vi "S4GUI_002.vi"(7 "Tab ObsEng":enum32{"Obs", "CCD modes", "Eng"}(tab)) -> ()   [LabVIEW 2018] (continued)
        n3103 = call-dynamic "Write Suffix.vi"("error in (no error)"=w6685, "Suffix"=w6751, "Interface in"=w6684) -> ("error out"=w6676:errorcluster, "Interface out"=w6679:refnum<class "Interface.lvclass">)  [unwired: 7 in]
        n3104 = call-dynamic "Write Suffix.vi"("error in (no error)"=w6649, "Suffix"=w6751, "Interface in"=w6650) -> ("error out"=w6658:errorcluster, "Interface out"=w6655:refnum<class "Interface.lvclass">)  [unwired: 7 in]
        n3105 = call-dynamic "Write ObsType.vi"("error in (no error)"=w6700, "ObsType"=w6729, "Interface in"=w6704) -> ("error out"=w6701:errorcluster, "Interface out"=w6705:refnum<class "Interface.lvclass">)  [unwired: 7 in]
        n3106 = call-dynamic "Write ObsType.vi"("error in (no error)"=w6624, "ObsType"=w6729, "Interface in"=w6627) -> ("error out"=w6625:errorcluster, "Interface out"=w6628:refnum<class "Interface.lvclass">)  [unwired: 7 in]
        n3107 = call-dynamic "Write ObsType.vi"("error in (no error)"=w6676, "ObsType"=w6729, "Interface in"=w6679) -> ("error out"=w6677:errorcluster, "Interface out"=w6680:refnum<class "Interface.lvclass">)  [unwired: 7 in]
        n3108 = call-dynamic "Write ObsType.vi"("error in (no error)"=w6658, "ObsType"=w6729, "Interface in"=w6655) -> ("error out"=w6657:errorcluster, "Interface out"=w6654:refnum<class "Interface.lvclass">)  [unwired: 7 in]
        n3109 = call-dynamic "Write Object.vi"("error in (no error)"=w6701, "Object"=w6730, "Interface in"=w6705) -> ("error out"=w6702:errorcluster, "Interface out"=w6706:refnum<class "Interface.lvclass">)  [unwired: 7 in]
        n3110 = call-dynamic "Write Object.vi"("error in (no error)"=w6677, "Object"=w6730, "Interface in"=w6680) -> ("error out"=w6678:errorcluster, "Interface out"=w6681:refnum<class "Interface.lvclass">)  [unwired: 7 in]
        n3111 = call-dynamic "Write Object.vi"("error in (no error)"=w6625, "Object"=w6730, "Interface in"=w6628) -> ("error out"=w6626:errorcluster, "Interface out"=w6629:refnum<class "Interface.lvclass">)  [unwired: 7 in]
        n3112 = call-dynamic "Write Object.vi"("error in (no error)"=w6657, "Object"=w6730, "Interface in"=w6654) -> ("error out"=w6656:errorcluster, "Interface out"=w6653:refnum<class "Interface.lvclass">)  [unwired: 7 in]
        n3113 = call-dynamic "Write Comments.vi"("error in (no error)"=w6626, "Comments"=w6723, "Interface in"=w6629) -> ("error out"=w6630:errorcluster, "Interface out"=w6631:refnum<class "Interface.lvclass">)  [unwired: 7 in]
        n3114 = call-dynamic "Write Comments.vi"("error in (no error)"=w6678, "Comments"=w6723, "Interface in"=w6681) -> ("error out"=w6682:errorcluster, "Interface out"=w6683:refnum<class "Interface.lvclass">)  [unwired: 7 in]
        n3115 = call-dynamic "Write Comments.vi"("error in (no error)"=w6656, "Comments"=w6723, "Interface in"=w6653) -> ("error out"=w6652:errorcluster, "Interface out"=w6651:refnum<class "Interface.lvclass">)  [unwired: 7 in]
        n3116 = call-dynamic "Write Comments.vi"("error in (no error)"=w6702, "Comments"=w6723, "Interface in"=w6706) -> ("error out"=w6707:errorcluster, "Interface out"=w6708:refnum<class "Interface.lvclass">)  [unwired: 7 in]
        n3117 = call-dynamic "Write Observer.vi"("error in (no error)"=w6630, "Observer"=w6728, "Interface in"=w6631) -> ("error out"=w6616:errorcluster, "Interface out"=w6615:refnum<class "Interface.lvclass">)  [unwired: 7 in]
        n3118 = call-dynamic "Write Observer.vi"("error in (no error)"=w6707, "Observer"=w6728, "Interface in"=w6708) -> ("error out"=w6693:errorcluster, "Interface out"=w6694:refnum<class "Interface.lvclass">)  [unwired: 7 in]
        n3119 = call-dynamic "Write Observer.vi"("error in (no error)"=w6682, "Observer"=w6728, "Interface in"=w6683) -> ("error out"=w6668:errorcluster, "Interface out"=w6667:refnum<class "Interface.lvclass">)  [unwired: 7 in]
        n3120 = call-dynamic "Write Observer.vi"("error in (no error)"=w6652, "Observer"=w6728, "Interface in"=w6651) -> ("error out"=w6642:errorcluster, "Interface out"=w6641:refnum<class "Interface.lvclass">)  [unwired: 7 in]
        n3121 = call-dynamic "Write Project ID.vi"("error in (no error)"=w6642, "Project ID"=w6727, "Interface in"=w6641) -> ("error out"=w6639:errorcluster, "Interface out"=w6640:refnum<class "Interface.lvclass">)  [unwired: 7 in]
        n3122 = call-dynamic "Write Project ID.vi"("error in (no error)"=w6668, "Project ID"=w6727, "Interface in"=w6667) -> ("error out"=w6665:errorcluster, "Interface out"=w6666:refnum<class "Interface.lvclass">)  [unwired: 7 in]
        n3123 = call-dynamic "Write Project ID.vi"("error in (no error)"=w6616, "Project ID"=w6727, "Interface in"=w6615) -> ("error out"=w6613:errorcluster, "Interface out"=w6614:refnum<class "Interface.lvclass">)  [unwired: 7 in]
        n3124 = call-dynamic "Write Project ID.vi"("error in (no error)"=w6693, "Project ID"=w6727, "Interface in"=w6694) -> ("error out"=w6691:errorcluster, "Interface out"=w6692:refnum<class "Interface.lvclass">)  [unwired: 7 in]
        n3125 = call-dynamic "Write Interface.vi"("error in (no error)"=w6665, "Interface.lvclass"=w6666, "Channel in"=w6674) -> ("error out"=w6672:errorcluster, "Channel out"=w6673:refnum<class "Channel.lvclass">)  [unwired: 7 in]
        n3126 = call-dynamic "Write Interface.vi"("error in (no error)"=w6691, "Interface.lvclass"=w6692, "Channel in"=w6703) -> ("error out"=w6697:errorcluster, "Channel out"=w6698:refnum<class "Channel.lvclass">)  [unwired: 7 in]
        n3127 = call-dynamic "Write Interface.vi"("error in (no error)"=w6639, "Interface.lvclass"=w6640, "Channel in"=w6660) -> ("error out"=w6646:errorcluster, "Channel out"=w6647:refnum<class "Channel.lvclass">)  [unwired: 7 in]
        n3128 = call-dynamic "Write Interface.vi"("error in (no error)"=w6613, "Interface.lvclass"=w6614, "Channel in"=w6622) -> ("error out"=w6620:errorcluster, "Channel out"=w6621:refnum<class "Channel.lvclass">)  [unwired: 7 in]
        n3129 = case shown="True" w6664 {
          tunnel: [w6805 w6816] -> w6689
          tunnel: [w6806 w6815] -> w6688
          tunnel: w6673 -> [w6806 w6808]
          tunnel: w6672 -> [w6805 w6807]
          frame False {
          }
          frame True {
            # "command SET SUFFIX"
            n3130 = call-dynamic "Read State Machine.vi"("error in (no error)"=w6807, "Device in"=w6808) -> ("error out"=w6809:errorcluster, "State Machine.lvclass"=w6813:refnum<class "State Machine.lvclass">, "Device out"=w6812:refnum<class "Channel.lvclass">)  [unwired: 7 in]
            n3131 = call-dynamic "Write State.vi"("error in (no error)"=w6809, "State"=300, "State Machine in"=w6813) -> ("error out"=w6810:errorcluster, "State Machine out"=w6814:refnum<class "State Machine.lvclass">)  [unwired: 7 in]
            n3132 = call-dynamic "Write State Machine.vi"("error in (no error)"=w6810, "State Machine.lvclass"=w6814, "Device in"=w6812) -> ("error out"=w6816:errorcluster, "Device out"=w6815:refnum<class "Channel.lvclass">)  [unwired: 7 in]
          }
        }
        n3133 = case shown="True" w6690 {
          tunnel: [w6818 w6822] -> w6714
          tunnel: [w6817 w6821] -> w6713
          tunnel: w6698 -> [w6818 w6820]
          tunnel: w6697 -> [w6817 w6819]
          frame False {
          }
          frame True {
            # "command SET SUFFIX"
            n3134 = call-dynamic "Read State Machine.vi"("error in (no error)"=w6819, "Device in"=w6820) -> ("error out"=w6828:errorcluster, "State Machine.lvclass"=w6824:refnum<class "State Machine.lvclass">, "Device out"=w6825:refnum<class "Channel.lvclass">)  [unwired: 7 in]
            n3135 = call-dynamic "Write State.vi"("error in (no error)"=w6828, "State"=300, "State Machine in"=w6824) -> ("error out"=w6827:errorcluster, "State Machine out"=w6823:refnum<class "State Machine.lvclass">)  [unwired: 7 in]
            n3136 = call-dynamic "Write State Machine.vi"("error in (no error)"=w6827, "State Machine.lvclass"=w6823, "Device in"=w6825) -> ("error out"=w6821:errorcluster, "Device out"=w6822:refnum<class "Channel.lvclass">)  [unwired: 7 in]
          }
        }
        n3137 = case shown="True" w6638 {
          tunnel: [w6793 w6804] -> w6663
          tunnel: [w6794 w6803] -> w6662
          tunnel: w6647 -> [w6794 w6796]
          tunnel: w6646 -> [w6793 w6795]
          frame False {
          }
          frame True {
            # "command SET SUFFIX"
            n3138 = call-dynamic "Read State Machine.vi"("error in (no error)"=w6795, "Device in"=w6796) -> ("error out"=w6797:errorcluster, "State Machine.lvclass"=w6801:refnum<class "State Machine.lvclass">, "Device out"=w6800:refnum<class "Channel.lvclass">)  [unwired: 7 in]
            n3139 = call-dynamic "Write State.vi"("error in (no error)"=w6797, "State"=300, "State Machine in"=w6801) -> ("error out"=w6798:errorcluster, "State Machine out"=w6802:refnum<class "State Machine.lvclass">)  [unwired: 7 in]
            n3140 = call-dynamic "Write State Machine.vi"("error in (no error)"=w6798, "State Machine.lvclass"=w6802, "Device in"=w6800) -> ("error out"=w6804:errorcluster, "Device out"=w6803:refnum<class "Channel.lvclass">)  [unwired: 7 in]
          }
        }
        n3141 = case shown="True" w6612 {
          tunnel: [w6782 w6786] -> w6636
          tunnel: [w6781 w6785] -> w6635
          tunnel: w6621 -> [w6782 w6784]
          tunnel: w6620 -> [w6781 w6783]
          frame False {
          }
          frame True {
            # "command SET SUFFIX"
            n3142 = call-dynamic "Read State Machine.vi"("error in (no error)"=w6783, "Device in"=w6784) -> ("error out"=w6792:errorcluster, "State Machine.lvclass"=w6788:refnum<class "State Machine.lvclass">, "Device out"=w6789:refnum<class "Channel.lvclass">)  [unwired: 7 in]
            n3143 = call-dynamic "Write State.vi"("error in (no error)"=w6792, "State"=300, "State Machine in"=w6788) -> ("error out"=w6791:errorcluster, "State Machine out"=w6787:refnum<class "State Machine.lvclass">)  [unwired: 7 in]
            n3144 = call-dynamic "Write State Machine.vi"("error in (no error)"=w6791, "State Machine.lvclass"=w6787, "Device in"=w6789) -> ("error out"=w6785:errorcluster, "Device out"=w6786:refnum<class "Channel.lvclass">)  [unwired: 7 in]
          }
        }
        n3145 = call-dynamic "Write Channel.vi"("error in (no error)"=w6713, "Channel.lvclass"=w6714, "Acquisition in"=w6715) -> ("error out"=w6778:errorcluster, "Acquisition out"=w6779:refnum<class "Acquisition.lvclass">)  [unwired: 7 in]
        n3146 = call-dynamic "Write Channel.vi"("error in (no error)"=w6689, "Channel.lvclass"=w6688, "Acquisition in"=w6687) -> ("error out"=w6773:errorcluster, "Acquisition out"=w6774:refnum<class "Acquisition.lvclass">)  [unwired: 7 in]
        n3147 = call-dynamic "Write Channel.vi"("error in (no error)"=w6663, "Channel.lvclass"=w6662, "Acquisition in"=w6661) -> ("error out"=w6762:errorcluster, "Acquisition out"=w6763:refnum<class "Acquisition.lvclass">)  [unwired: 7 in]
        n3148 = call-dynamic "Write Channel.vi"("error in (no error)"=w6635, "Channel.lvclass"=w6636, "Acquisition in"=w6637) -> ("error out"=w6760:errorcluster, "Acquisition out"=w6761:refnum<class "Acquisition.lvclass">)  [unwired: 7 in]
        n3149 = call-dynamic "Write AcquisitionA.vi"("error in (no error)"=w6778, "Acquisition.lvclass"=w6779, "S4ACS_GUI in"=w6780) -> ("error out"=w6768:errorcluster, "S4ACS_GUI out"=w6772:refnum<class "S4GUI.lvclass">)  [unwired: 7 in]
        n3150 = call "Write AcquisitionB.vi"("error in (no error)"=w6773, "Acquisition.lvclass"=w6774, "S4ACS_GUI in"=w6772) -> ("error out"=w6767:errorcluster, "S4ACS_GUI out"=w6771:refnum<class "S4GUI.lvclass">)  [unwired: 7 in]
        n3151 = call-dynamic "Write AcquisitionC.vi"("error in (no error)"=w6762, "Acquisition.lvclass"=w6763, "S4ACS_GUI in"=w6771) -> ("error out"=w6766:errorcluster, "S4ACS_GUI out"=w6770:refnum<class "S4GUI.lvclass">)  [unwired: 7 in]
        n3152 = call-dynamic "Write AcquisitionD.vi"("error in (no error)"=w6760, "Acquisition.lvclass"=w6761, "S4ACS_GUI in"=w6770) -> ("error out"=w6765:errorcluster, "S4ACS_GUI out"=w6769:refnum<class "S4GUI.lvclass">)  [unwired: 7 in]
        n3153 = Merge Errors(w6768, w6767, w6766, w6765) -> (w6764:errorcluster)
        n3154 = call "Write cfg file.vi"("error in (no error)"=w6764, "cfg file"="lastsaved.cfg", "S4ACS_GUI in"=w6769) -> ("error out"=w6776:errorcluster, "S4ACS_GUI out"=w6775:refnum<class "S4GUI.lvclass">)  [unwired: 7 in]
      }
      event "Object_sflat", "Object_dark", "Object_zero", "Object_dflat", "Object_focus", "Object_obj": Value Change {
        n3155 = event-data() -> ("NewVal"=w6854:string)  [unwired: 1 in, 5 out]
        n3156 = stacked-sequence {
          seq-local: [w6884 _ _ _] -> [_ w6948 _ _]
          seq-local: [w6883 _ _ _] -> [_ w6947 _ _]
          seq-local: [_ w6946 _ _] -> [_ _ w6997 _]
          seq-local: [_ w6945 _ _] -> [_ _ w6996 _]
          seq-local: [_ _ w6995 _] -> [_ _ _ w7046]
          seq-local: [_ _ w6994 _] -> [_ _ _ w7045]
          tunnel: w6861 -> [w6896 _ _ _]
          tunnel: w6862 -> [w6895 _ _ _]
          tunnel: [_ _ _ w7044] -> w6856
          tunnel: [_ _ _ w7043] -> w6855
          tunnel: w6860 -> [w6882 w6944 w6993 w7042]
          tunnel: w6859 -> [w6881 w6943 w6979 w7028]
          tunnel: w6857 -> [w6880 w6929 w6978 w7027]
          tunnel: w6854 -> [w6879 w6928 w6977 w7026]
          tunnel: w6858 -> [w6878 w6927 w6976 w7025]
          frame #0 {
            # "observer"
            # "comment"
            # "object"
            # "suffix"
            # "obsType"
            n3157 = call-dynamic "Read AcquisitionA.vi"("error in (no error)"=w6896, "S4ACS_GUI in"=w6895) -> ("error out"=w6894:errorcluster, "Acquisition.lvclass"=w6893:refnum<class "Acquisition.lvclass">, "S4ACS_GUI out"=w6888:refnum<class "S4GUI.lvclass">)  [unwired: 7 in]
            n3158 = call-dynamic "Read Channel.vi"("error in (no error)"=w6894, "Acquisition in"=w6893) -> ("error out"=w6864:errorcluster, "Channel.lvclass"=w6867:refnum<class "Channel.lvclass">, "Acquisition out"=w6887:refnum<class "Acquisition.lvclass">)  [unwired: 7 in]
            n3159 = local read "Filter1"() -> (w6865:u8)
            n3160 = call-dynamic "Write Filter.vi"("error in (no error)"=w6864, "Filter"=w6865, "Channel in"=w6867) -> ("error out"=w6863:errorcluster, "Channel out"=w6866:refnum<class "Channel.lvclass">)  [unwired: 7 in]
            n3161 = call-dynamic "Read Interface.vi"("error in (no error)"=w6863, "Channel in"=w6866) -> ("error out"=w6874:errorcluster, "Interface.lvclass"=w6875:refnum<class "Interface.lvclass">, "Channel out"=w6892:refnum<class "Channel.lvclass">)  [unwired: 7 in]
            n3162 = call-dynamic "Write Suffix.vi"("error in (no error)"=w6874, "Suffix"=w6882, "Interface in"=w6875) -> ("error out"=w6899:errorcluster, "Interface out"=w6891:refnum<class "Interface.lvclass">)  [unwired: 7 in]
            n3163 = call-dynamic "Write ObsType.vi"("error in (no error)"=w6899, "ObsType"=w6880, "Interface in"=w6891) -> ("error out"=w6898:errorcluster, "Interface out"=w6890:refnum<class "Interface.lvclass">)  [unwired: 7 in]
            n3164 = call-dynamic "Write Object.vi"("error in (no error)"=w6898, "Object"=w6879, "Interface in"=w6890) -> ("error out"=w6897:errorcluster, "Interface out"=w6889:refnum<class "Interface.lvclass">)  [unwired: 7 in]
            n3165 = call-dynamic "Write Comments.vi"("error in (no error)"=w6897, "Comments"=w6881, "Interface in"=w6889) -> ("error out"=w6877:errorcluster, "Interface out"=w6876:refnum<class "Interface.lvclass">)  [unwired: 7 in]
            n3166 = call-dynamic "Write Observer.vi"("error in (no error)"=w6877, "Observer"=w6878, "Interface in"=w6876) -> ("error out"=w6872:errorcluster, "Interface out"=w6873:refnum<class "Interface.lvclass">)  [unwired: 7 in]
            n3167 = call-dynamic "Write Interface.vi"("error in (no error)"=w6872, "Interface.lvclass"=w6873, "Channel in"=w6892) -> ("error out"=w6869:errorcluster, "Channel out"=w6871:refnum<class "Channel.lvclass">)  [unwired: 7 in]
            n3168 = disable-structure shown="Enabled" {
              disable-tunnel: w6871 -> [w6909 w6911]
              disable-tunnel: [w6907 w6911] -> w6870
              disable-tunnel: w6869 -> [w6906 w6910]
              disable-tunnel: [w6901 w6910] -> w6868
              frame Disabled {
                n3169 = call-dynamic "Read State Machine.vi"("error in (no error)"=w6906, "Device in"=w6909) -> ("error out"=w6905:errorcluster, "State Machine.lvclass"=w6903:refnum<class "State Machine.lvclass">, "Device out"=w6908:refnum<class "Channel.lvclass">)  [unwired: 7 in]
                n3170 = call "Next State.vi"("error in (no error)"=w6905, "New_State"=12, "State Machine in"=w6903) -> ("error out"=w6904:errorcluster, "State Machine out"=w6902:refnum<class "State Machine.lvclass">)  [unwired: 7 in]
                n3171 = call-dynamic "Write State Machine.vi"("error in (no error)"=w6904, "State Machine.lvclass"=w6902, "Device in"=w6908) -> ("error out"=w6901:errorcluster, "Device out"=w6907:refnum<class "Channel.lvclass">)  [unwired: 7 in]
              }
              frame Enabled {
              }
            }
            n3172 = call-dynamic "Write Channel.vi"("error in (no error)"=w6868, "Channel.lvclass"=w6870, "Acquisition in"=w6887) -> ("error out"=w6885:errorcluster, "Acquisition out"=w6886:refnum<class "Acquisition.lvclass">)  [unwired: 7 in]
            n3173 = call-dynamic "Write AcquisitionA.vi"("error in (no error)"=w6885, "Acquisition.lvclass"=w6886, "S4ACS_GUI in"=w6888) -> ("error out"=w6883:errorcluster, "S4ACS_GUI out"=w6884:refnum<class "S4GUI.lvclass">)  [unwired: 7 in]
          }
          frame #1 {
            # "object"
            # "suffix"
            # "obsType"
            n3174 = call "Read AcquisitionB.vi"("error in (no error)"=w6947, "S4ACS_GUI in"=w6948) -> ("error out"=w6933:errorcluster, "Acquisition.lvclass"=w6934:refnum<class "Acquisition.lvclass">, "S4ACS_GUI out"=w6939:refnum<class "S4GUI.lvclass">)  [unwired: 7 in]
            n3175 = call-dynamic "Read Channel.vi"("error in (no error)"=w6933, "Acquisition in"=w6934) -> ("error out"=w6913:errorcluster, "Channel.lvclass"=w6915:refnum<class "Channel.lvclass">, "Acquisition out"=w6940:refnum<class "Acquisition.lvclass">)  [unwired: 7 in]
            n3176 = local read "Filter2"() -> (w6916:u8)
            n3177 = call-dynamic "Write Filter.vi"("error in (no error)"=w6913, "Filter"=w6916, "Channel in"=w6915) -> ("error out"=w6912:errorcluster, "Channel out"=w6914:refnum<class "Channel.lvclass">)  [unwired: 7 in]
            n3178 = call-dynamic "Read Interface.vi"("error in (no error)"=w6912, "Channel in"=w6914) -> ("error out"=w6921:errorcluster, "Interface.lvclass"=w6922:refnum<class "Interface.lvclass">, "Channel out"=w6935:refnum<class "Channel.lvclass">)  [unwired: 7 in]
            n3179 = call-dynamic "Write Suffix.vi"("error in (no error)"=w6921, "Suffix"=w6944, "Interface in"=w6922) -> ("error out"=w6930:errorcluster, "Interface out"=w6936:refnum<class "Interface.lvclass">)  [unwired: 7 in]
            n3180 = call-dynamic "Write ObsType.vi"("error in (no error)"=w6930, "ObsType"=w6929, "Interface in"=w6936) -> ("error out"=w6931:errorcluster, "Interface out"=w6937:refnum<class "Interface.lvclass">)  [unwired: 7 in]
            n3181 = call-dynamic "Write Object.vi"("error in (no error)"=w6931, "Object"=w6928, "Interface in"=w6937) -> ("error out"=w6932:errorcluster, "Interface out"=w6938:refnum<class "Interface.lvclass">)  [unwired: 7 in]
            n3182 = call-dynamic "Write Comments.vi"("error in (no error)"=w6932, "Comments"=w6943, "Interface in"=w6938) -> ("error out"=w6924:errorcluster, "Interface out"=w6923:refnum<class "Interface.lvclass">)  [unwired: 7 in]
            n3183 = call-dynamic "Write Observer.vi"("error in (no error)"=w6924, "Observer"=w6927, "Interface in"=w6923) -> ("error out"=w6925:errorcluster, "Interface out"=w6926:refnum<class "Interface.lvclass">)  [unwired: 7 in]
            n3184 = call-dynamic "Write Interface.vi"("error in (no error)"=w6925, "Interface.lvclass"=w6926, "Channel in"=w6935) -> ("error out"=w6919:errorcluster, "Channel out"=w6920:refnum<class "Channel.lvclass">)  [unwired: 7 in]
            n3185 = disable-structure shown="Enabled" {
              disable-tunnel: w6920 -> [w6953 w6960]
              disable-tunnel: w6919 -> [w6952 w6959]
              disable-tunnel: [w6950 w6960] -> w6918
              disable-tunnel: [w6949 w6959] -> w6917
              frame Disabled {
                n3186 = call-dynamic "Read State Machine.vi"("error in (no error)"=w6952, "Device in"=w6953) -> ("error out"=w6958:errorcluster, "State Machine.lvclass"=w6956:refnum<class "State Machine.lvclass">, "Device out"=w6951:refnum<class "Channel.lvclass">)  [unwired: 7 in]
                n3187 = call "Next State.vi"("error in (no error)"=w6958, "New_State"=12, "State Machine in"=w6956) -> ("error out"=w6957:errorcluster, "State Machine out"=w6955:refnum<class "State Machine.lvclass">)  [unwired: 7 in]
                n3188 = call-dynamic "Write State Machine.vi"("error in (no error)"=w6957, "State Machine.lvclass"=w6955, "Device in"=w6951) -> ("error out"=w6949:errorcluster, "Device out"=w6950:refnum<class "Channel.lvclass">)  [unwired: 7 in]
              }
              frame Enabled {
              }
            }
            n3189 = call-dynamic "Write Channel.vi"("error in (no error)"=w6917, "Channel.lvclass"=w6918, "Acquisition in"=w6940) -> ("error out"=w6942:errorcluster, "Acquisition out"=w6941:refnum<class "Acquisition.lvclass">)  [unwired: 7 in]
            n3190 = call "Write AcquisitionB.vi"("error in (no error)"=w6942, "Acquisition.lvclass"=w6941, "S4ACS_GUI in"=w6939) -> ("error out"=w6945:errorcluster, "S4ACS_GUI out"=w6946:refnum<class "S4GUI.lvclass">)  [unwired: 7 in]
          }
          frame #2 {
            # "object"
            # "suffix"
            # "obsType"
            n3191 = call-dynamic "Read AcquisitionC.vi"("error in (no error)"=w6996, "S4ACS_GUI in"=w6997) -> ("error out"=w6989:errorcluster, "Acquisition.lvclass"=w6988:refnum<class "Acquisition.lvclass">, "S4ACS_GUI out"=w6983:refnum<class "S4GUI.lvclass">)  [unwired: 7 in]
            n3192 = call-dynamic "Read Channel.vi"("error in (no error)"=w6989, "Acquisition in"=w6988) -> ("error out"=w6962:errorcluster, "Channel.lvclass"=w6964:refnum<class "Channel.lvclass">, "Acquisition out"=w6982:refnum<class "Acquisition.lvclass">)  [unwired: 7 in]
            n3193 = local read "Filter3"() -> (w6965:u8)
            n3194 = call-dynamic "Write Filter.vi"("error in (no error)"=w6962, "Filter"=w6965, "Channel in"=w6964) -> ("error out"=w6961:errorcluster, "Channel out"=w6963:refnum<class "Channel.lvclass">)  [unwired: 7 in]
            n3195 = call-dynamic "Read Interface.vi"("error in (no error)"=w6961, "Channel in"=w6963) -> ("error out"=w6974:errorcluster, "Interface.lvclass"=w6975:refnum<class "Interface.lvclass">, "Channel out"=w6987:refnum<class "Channel.lvclass">)  [unwired: 7 in]
            n3196 = call-dynamic "Write Suffix.vi"("error in (no error)"=w6974, "Suffix"=w6993, "Interface in"=w6975) -> ("error out"=w6992:errorcluster, "Interface out"=w6986:refnum<class "Interface.lvclass">)  [unwired: 7 in]
            n3197 = call-dynamic "Write ObsType.vi"("error in (no error)"=w6992, "ObsType"=w6978, "Interface in"=w6986) -> ("error out"=w6991:errorcluster, "Interface out"=w6985:refnum<class "Interface.lvclass">)  [unwired: 7 in]
            n3198 = call-dynamic "Write Object.vi"("error in (no error)"=w6991, "Object"=w6977, "Interface in"=w6985) -> ("error out"=w6990:errorcluster, "Interface out"=w6984:refnum<class "Interface.lvclass">)  [unwired: 7 in]
            n3199 = call-dynamic "Write Comments.vi"("error in (no error)"=w6990, "Comments"=w6979, "Interface in"=w6984) -> ("error out"=w6971:errorcluster, "Interface out"=w6970:refnum<class "Interface.lvclass">)  [unwired: 7 in]
            n3200 = call-dynamic "Write Observer.vi"("error in (no error)"=w6971, "Observer"=w6976, "Interface in"=w6970) -> ("error out"=w6972:errorcluster, "Interface out"=w6973:refnum<class "Interface.lvclass">)  [unwired: 7 in]
            n3201 = call-dynamic "Write Interface.vi"("error in (no error)"=w6972, "Interface.lvclass"=w6973, "Channel in"=w6987) -> ("error out"=w6968:errorcluster, "Channel out"=w6969:refnum<class "Channel.lvclass">)  [unwired: 7 in]
            n3202 = disable-structure shown="Enabled" {
              disable-tunnel: w6969 -> [w7004 w7009]
              disable-tunnel: w6968 -> [w7003 w7008]
              disable-tunnel: [w7001 w7009] -> w6967
              disable-tunnel: [w6998 w7008] -> w6966
              frame Disabled {
                n3203 = call-dynamic "Read State Machine.vi"("error in (no error)"=w7003, "Device in"=w7004) -> ("error out"=w7007:errorcluster, "State Machine.lvclass"=w7000:refnum<class "State Machine.lvclass">, "Device out"=w7002:refnum<class "Channel.lvclass">)  [unwired: 7 in]
                n3204 = call "Next State.vi"("error in (no error)"=w7007, "New_State"=12, "State Machine in"=w7000) -> ("error out"=w7006:errorcluster, "State Machine out"=w6999:refnum<class "State Machine.lvclass">)  [unwired: 7 in]
                n3205 = call-dynamic "Write State Machine.vi"("error in (no error)"=w7006, "State Machine.lvclass"=w6999, "Device in"=w7002) -> ("error out"=w6998:errorcluster, "Device out"=w7001:refnum<class "Channel.lvclass">)  [unwired: 7 in]
              }
              frame Enabled {
              }
            }
            n3206 = call-dynamic "Write Channel.vi"("error in (no error)"=w6966, "Channel.lvclass"=w6967, "Acquisition in"=w6982) -> ("error out"=w6980:errorcluster, "Acquisition out"=w6981:refnum<class "Acquisition.lvclass">)  [unwired: 7 in]
            n3207 = call-dynamic "Write AcquisitionC.vi"("error in (no error)"=w6980, "Acquisition.lvclass"=w6981, "S4ACS_GUI in"=w6983) -> ("error out"=w6994:errorcluster, "S4ACS_GUI out"=w6995:refnum<class "S4GUI.lvclass">)  [unwired: 7 in]
          }
          frame #3 {
            # "object"
            # "suffix"
            # "obsType"
            n3208 = call-dynamic "Read AcquisitionD.vi"("error in (no error)"=w7045, "S4ACS_GUI in"=w7046) -> ("error out"=w7038:errorcluster, "Acquisition.lvclass"=w7037:refnum<class "Acquisition.lvclass">, "S4ACS_GUI out"=w7032:refnum<class "S4GUI.lvclass">)  [unwired: 7 in]
            n3209 = call-dynamic "Read Channel.vi"("error in (no error)"=w7038, "Acquisition in"=w7037) -> ("error out"=w7011:errorcluster, "Channel.lvclass"=w7013:refnum<class "Channel.lvclass">, "Acquisition out"=w7031:refnum<class "Acquisition.lvclass">)  [unwired: 7 in]
            n3210 = local read "Filter4"() -> (w7014:u8)
            n3211 = call-dynamic "Write Filter.vi"("error in (no error)"=w7011, "Filter"=w7014, "Channel in"=w7013) -> ("error out"=w7010:errorcluster, "Channel out"=w7012:refnum<class "Channel.lvclass">)  [unwired: 7 in]
            n3212 = call-dynamic "Read Interface.vi"("error in (no error)"=w7010, "Channel in"=w7012) -> ("error out"=w7023:errorcluster, "Interface.lvclass"=w7024:refnum<class "Interface.lvclass">, "Channel out"=w7036:refnum<class "Channel.lvclass">)  [unwired: 7 in]
            n3213 = call-dynamic "Write Suffix.vi"("error in (no error)"=w7023, "Suffix"=w7042, "Interface in"=w7024) -> ("error out"=w7041:errorcluster, "Interface out"=w7035:refnum<class "Interface.lvclass">)  [unwired: 7 in]
            n3214 = call-dynamic "Write ObsType.vi"("error in (no error)"=w7041, "ObsType"=w7027, "Interface in"=w7035) -> ("error out"=w7040:errorcluster, "Interface out"=w7034:refnum<class "Interface.lvclass">)  [unwired: 7 in]
            n3215 = call-dynamic "Write Object.vi"("error in (no error)"=w7040, "Object"=w7026, "Interface in"=w7034) -> ("error out"=w7039:errorcluster, "Interface out"=w7033:refnum<class "Interface.lvclass">)  [unwired: 7 in]
            n3216 = call-dynamic "Write Comments.vi"("error in (no error)"=w7039, "Comments"=w7028, "Interface in"=w7033) -> ("error out"=w7022:errorcluster, "Interface out"=w7021:refnum<class "Interface.lvclass">)  [unwired: 7 in]
            n3217 = call-dynamic "Write Observer.vi"("error in (no error)"=w7022, "Observer"=w7025, "Interface in"=w7021) -> ("error out"=w7020:errorcluster, "Interface out"=w7019:refnum<class "Interface.lvclass">)  [unwired: 7 in]
            n3218 = call-dynamic "Write Interface.vi"("error in (no error)"=w7020, "Interface.lvclass"=w7019, "Channel in"=w7036) -> ("error out"=w7016:errorcluster, "Channel out"=w7018:refnum<class "Channel.lvclass">)  [unwired: 7 in]
            n3219 = disable-structure shown="Enabled" {
              disable-tunnel: w7018 -> [w7053 w7058]
              disable-tunnel: [w7051 w7058] -> w7017
              disable-tunnel: w7016 -> [w7050 w7057]
              disable-tunnel: [w7049 w7057] -> w7015
              frame Disabled {
                n3220 = call-dynamic "Read State Machine.vi"("error in (no error)"=w7050, "Device in"=w7053) -> ("error out"=w7056:errorcluster, "State Machine.lvclass"=w7048:refnum<class "State Machine.lvclass">, "Device out"=w7052:refnum<class "Channel.lvclass">)  [unwired: 7 in]
                n3221 = call "Next State.vi"("error in (no error)"=w7056, "New_State"=12, "State Machine in"=w7048) -> ("error out"=w7055:errorcluster, "State Machine out"=w7047:refnum<class "State Machine.lvclass">)  [unwired: 7 in]
                n3222 = call-dynamic "Write State Machine.vi"("error in (no error)"=w7055, "State Machine.lvclass"=w7047, "Device in"=w7052) -> ("error out"=w7049:errorcluster, "Device out"=w7051:refnum<class "Channel.lvclass">)  [unwired: 7 in]
              }
              frame Enabled {
              }
            }
            n3223 = call-dynamic "Write Channel.vi"("error in (no error)"=w7015, "Channel.lvclass"=w7017, "Acquisition in"=w7031) -> ("error out"=w7029:errorcluster, "Acquisition out"=w7030:refnum<class "Acquisition.lvclass">)  [unwired: 7 in]
            n3224 = call-dynamic "Write AcquisitionD.vi"("error in (no error)"=w7029, "Acquisition.lvclass"=w7030, "S4ACS_GUI in"=w7032) -> ("error out"=w7043:errorcluster, "S4ACS_GUI out"=w7044:refnum<class "S4GUI.lvclass">)  [unwired: 7 in]
          }
        }
      }
      event "DFLAT Comments", "SFLAT Comments", "DARK Comments", "ZERO Comments", "FOCUS Comments", "OBJECT Comments": Value Change {
        n3225 = event-data() -> ("NewVal"=w7059:string)  [unwired: 1 in, 5 out]
        n3226 = disable-structure shown="Enabled" {
          disable-tunnel: w7067 -> [w7076 w7250]
          disable-tunnel: w7066 -> [w7075 w7249]
          disable-tunnel: w7065 -> [w7074 _]
          disable-tunnel: w7064 -> [w7073 _]
          disable-tunnel: w7063 -> [w7072 _]
          disable-tunnel: w7062 -> [w7071 _]
          disable-tunnel: [w7070 w7250] -> w7061
          disable-tunnel: [w7069 w7249] -> w7060
          disable-tunnel: w7059 -> [w7068 _]
          frame Disabled {
            n3227 = stacked-sequence {
              seq-local: [w7104 _ _ _] -> [_ w7162 _ _]
              seq-local: [w7103 _ _ _] -> [_ w7161 _ _]
              seq-local: [_ w7160 _ _] -> [_ _ w7205 _]
              seq-local: [_ w7159 _ _] -> [_ _ w7204 _]
              seq-local: [_ _ w7203 _] -> [_ _ _ w7248]
              seq-local: [_ _ w7202 _] -> [_ _ _ w7247]
              tunnel: w7075 -> [w7116 _ _ _]
              tunnel: w7076 -> [w7115 _ _ _]
              tunnel: [_ _ _ w7246] -> w7070
              tunnel: [_ _ _ w7245] -> w7069
              tunnel: w7073 -> [w7102 w7158 w7201 w7244]
              tunnel: w7068 -> [w7101 w7157 w7187 w7230]
              tunnel: w7071 -> [w7100 w7143 w7186 w7229]
              tunnel: w7074 -> [w7099 w7142 w7185 w7228]
              tunnel: w7072 -> [w7098 w7141 w7184 w7227]
              frame #0 {
                # "observer"
                # "comment"
                # "object"
                # "suffix"
                # "obsType"
                n3228 = call-dynamic "Read AcquisitionA.vi"("error in (no error)"=w7116, "S4ACS_GUI in"=w7115) -> ("error out"=w7114:errorcluster, "Acquisition.lvclass"=w7113:refnum<class "Acquisition.lvclass">, "S4ACS_GUI out"=w7108:refnum<class "S4GUI.lvclass">)  [unwired: 7 in]
                n3229 = call-dynamic "Read Channel.vi"("error in (no error)"=w7114, "Acquisition in"=w7113) -> ("error out"=w7078:errorcluster, "Channel.lvclass"=w7081:refnum<class "Channel.lvclass">, "Acquisition out"=w7107:refnum<class "Acquisition.lvclass">)  [unwired: 7 in]
                n3230 = local read "Filter1"() -> (w7079:u8)
                n3231 = call-dynamic "Write Filter.vi"("error in (no error)"=w7078, "Filter"=w7079, "Channel in"=w7081) -> ("error out"=w7077:errorcluster, "Channel out"=w7080:refnum<class "Channel.lvclass">)  [unwired: 7 in]
                n3232 = call-dynamic "Read Interface.vi"("error in (no error)"=w7077, "Channel in"=w7080) -> ("error out"=w7094:errorcluster, "Interface.lvclass"=w7095:refnum<class "Interface.lvclass">, "Channel out"=w7112:refnum<class "Channel.lvclass">)  [unwired: 7 in]
                n3233 = call-dynamic "Write Suffix.vi"("error in (no error)"=w7094, "Suffix"=w7102, "Interface in"=w7095) -> ("error out"=w7119:errorcluster, "Interface out"=w7111:refnum<class "Interface.lvclass">)  [unwired: 7 in]
                n3234 = call-dynamic "Write ObsType.vi"("error in (no error)"=w7119, "ObsType"=w7100, "Interface in"=w7111) -> ("error out"=w7118:errorcluster, "Interface out"=w7110:refnum<class "Interface.lvclass">)  [unwired: 7 in]
                n3235 = call-dynamic "Write Object.vi"("error in (no error)"=w7118, "Object"=w7099, "Interface in"=w7110) -> ("error out"=w7117:errorcluster, "Interface out"=w7109:refnum<class "Interface.lvclass">)  [unwired: 7 in]
                n3236 = call-dynamic "Write Comments.vi"("error in (no error)"=w7117, "Comments"=w7101, "Interface in"=w7109) -> ("error out"=w7097:errorcluster, "Interface out"=w7096:refnum<class "Interface.lvclass">)  [unwired: 7 in]
                n3237 = call-dynamic "Write Observer.vi"("error in (no error)"=w7097, "Observer"=w7098, "Interface in"=w7096) -> ("error out"=w7092:errorcluster, "Interface out"=w7093:refnum<class "Interface.lvclass">)  [unwired: 7 in]
                n3238 = call-dynamic "Write Interface.vi"("error in (no error)"=w7092, "Interface.lvclass"=w7093, "Channel in"=w7112) -> ("error out"=w7088:errorcluster, "Channel out"=w7091:refnum<class "Channel.lvclass">)  [unwired: 7 in]
                n3239 = call-dynamic "Read State Machine.vi"("error in (no error)"=w7088, "Device in"=w7091) -> ("error out"=w7087:errorcluster, "State Machine.lvclass"=w7085:refnum<class "State Machine.lvclass">, "Device out"=w7090:refnum<class "Channel.lvclass">)  [unwired: 7 in]
                n3240 = call "Next State.vi"("error in (no error)"=w7087, "New_State"=12, "State Machine in"=w7085) -> ("error out"=w7086:errorcluster, "State Machine out"=w7084:refnum<class "State Machine.lvclass">)  [unwired: 7 in]
                n3241 = call-dynamic "Write State Machine.vi"("error in (no error)"=w7086, "State Machine.lvclass"=w7084, "Device in"=w7090) -> ("error out"=w7083:errorcluster, "Device out"=w7089:refnum<class "Channel.lvclass">)  [unwired: 7 in]
                n3242 = call-dynamic "Write Channel.vi"("error in (no error)"=w7083, "Channel.lvclass"=w7089, "Acquisition in"=w7107) -> ("error out"=w7105:errorcluster, "Acquisition out"=w7106:refnum<class "Acquisition.lvclass">)  [unwired: 7 in]
                n3243 = call-dynamic "Write AcquisitionA.vi"("error in (no error)"=w7105, "Acquisition.lvclass"=w7106, "S4ACS_GUI in"=w7108) -> ("error out"=w7103:errorcluster, "S4ACS_GUI out"=w7104:refnum<class "S4GUI.lvclass">)  [unwired: 7 in]
              }
              frame #1 {
                # "object"
                # "suffix"
                # "obsType"
                n3244 = call "Read AcquisitionB.vi"("error in (no error)"=w7161, "S4ACS_GUI in"=w7162) -> ("error out"=w7147:errorcluster, "Acquisition.lvclass"=w7148:refnum<class "Acquisition.lvclass">, "S4ACS_GUI out"=w7153:refnum<class "S4GUI.lvclass">)  [unwired: 7 in]
                n3245 = call-dynamic "Read Channel.vi"("error in (no error)"=w7147, "Acquisition in"=w7148) -> ("error out"=w7121:errorcluster, "Channel.lvclass"=w7123:refnum<class "Channel.lvclass">, "Acquisition out"=w7154:refnum<class "Acquisition.lvclass">)  [unwired: 7 in]
                n3246 = local read "Filter2"() -> (w7124:u8)
                n3247 = call-dynamic "Write Filter.vi"("error in (no error)"=w7121, "Filter"=w7124, "Channel in"=w7123) -> ("error out"=w7120:errorcluster, "Channel out"=w7122:refnum<class "Channel.lvclass">)  [unwired: 7 in]
                n3248 = call-dynamic "Read Interface.vi"("error in (no error)"=w7120, "Channel in"=w7122) -> ("error out"=w7135:errorcluster, "Interface.lvclass"=w7136:refnum<class "Interface.lvclass">, "Channel out"=w7149:refnum<class "Channel.lvclass">)  [unwired: 7 in]
                n3249 = call-dynamic "Write Suffix.vi"("error in (no error)"=w7135, "Suffix"=w7158, "Interface in"=w7136) -> ("error out"=w7144:errorcluster, "Interface out"=w7150:refnum<class "Interface.lvclass">)  [unwired: 7 in]
                n3250 = call-dynamic "Write ObsType.vi"("error in (no error)"=w7144, "ObsType"=w7143, "Interface in"=w7150) -> ("error out"=w7145:errorcluster, "Interface out"=w7151:refnum<class "Interface.lvclass">)  [unwired: 7 in]
                n3251 = call-dynamic "Write Object.vi"("error in (no error)"=w7145, "Object"=w7142, "Interface in"=w7151) -> ("error out"=w7146:errorcluster, "Interface out"=w7152:refnum<class "Interface.lvclass">)  [unwired: 7 in]
                n3252 = call-dynamic "Write Comments.vi"("error in (no error)"=w7146, "Comments"=w7157, "Interface in"=w7152) -> ("error out"=w7138:errorcluster, "Interface out"=w7137:refnum<class "Interface.lvclass">)  [unwired: 7 in]
                n3253 = call-dynamic "Write Observer.vi"("error in (no error)"=w7138, "Observer"=w7141, "Interface in"=w7137) -> ("error out"=w7139:errorcluster, "Interface out"=w7140:refnum<class "Interface.lvclass">)  [unwired: 7 in]
                n3254 = call-dynamic "Write Interface.vi"("error in (no error)"=w7139, "Interface.lvclass"=w7140, "Channel in"=w7149) -> ("error out"=w7128:errorcluster, "Channel out"=w7129:refnum<class "Channel.lvclass">)  [unwired: 7 in]
                n3255 = call-dynamic "Read State Machine.vi"("error in (no error)"=w7128, "Device in"=w7129) -> ("error out"=w7134:errorcluster, "State Machine.lvclass"=w7132:refnum<class "State Machine.lvclass">, "Device out"=w7127:refnum<class "Channel.lvclass">)  [unwired: 7 in]
                n3256 = call "Next State.vi"("error in (no error)"=w7134, "New_State"=12, "State Machine in"=w7132) -> ("error out"=w7133:errorcluster, "State Machine out"=w7131:refnum<class "State Machine.lvclass">)  [unwired: 7 in]
                n3257 = call-dynamic "Write State Machine.vi"("error in (no error)"=w7133, "State Machine.lvclass"=w7131, "Device in"=w7127) -> ("error out"=w7125:errorcluster, "Device out"=w7126:refnum<class "Channel.lvclass">)  [unwired: 7 in]
                n3258 = call-dynamic "Write Channel.vi"("error in (no error)"=w7125, "Channel.lvclass"=w7126, "Acquisition in"=w7154) -> ("error out"=w7156:errorcluster, "Acquisition out"=w7155:refnum<class "Acquisition.lvclass">)  [unwired: 7 in]
                n3259 = call "Write AcquisitionB.vi"("error in (no error)"=w7156, "Acquisition.lvclass"=w7155, "S4ACS_GUI in"=w7153) -> ("error out"=w7159:errorcluster, "S4ACS_GUI out"=w7160:refnum<class "S4GUI.lvclass">)  [unwired: 7 in]
              }
              frame #2 {
                # "object"
                # "suffix"
                # "obsType"
                n3260 = call-dynamic "Read AcquisitionC.vi"("error in (no error)"=w7204, "S4ACS_GUI in"=w7205) -> ("error out"=w7197:errorcluster, "Acquisition.lvclass"=w7196:refnum<class "Acquisition.lvclass">, "S4ACS_GUI out"=w7191:refnum<class "S4GUI.lvclass">)  [unwired: 7 in]
                n3261 = call-dynamic "Read Channel.vi"("error in (no error)"=w7197, "Acquisition in"=w7196) -> ("error out"=w7164:errorcluster, "Channel.lvclass"=w7166:refnum<class "Channel.lvclass">, "Acquisition out"=w7190:refnum<class "Acquisition.lvclass">)  [unwired: 7 in]
                n3262 = local read "Filter3"() -> (w7167:u8)
                n3263 = call-dynamic "Write Filter.vi"("error in (no error)"=w7164, "Filter"=w7167, "Channel in"=w7166) -> ("error out"=w7163:errorcluster, "Channel out"=w7165:refnum<class "Channel.lvclass">)  [unwired: 7 in]
                n3264 = call-dynamic "Read Interface.vi"("error in (no error)"=w7163, "Channel in"=w7165) -> ("error out"=w7182:errorcluster, "Interface.lvclass"=w7183:refnum<class "Interface.lvclass">, "Channel out"=w7195:refnum<class "Channel.lvclass">)  [unwired: 7 in]
                n3265 = call-dynamic "Write Suffix.vi"("error in (no error)"=w7182, "Suffix"=w7201, "Interface in"=w7183) -> ("error out"=w7200:errorcluster, "Interface out"=w7194:refnum<class "Interface.lvclass">)  [unwired: 7 in]
                n3266 = call-dynamic "Write ObsType.vi"("error in (no error)"=w7200, "ObsType"=w7186, "Interface in"=w7194) -> ("error out"=w7199:errorcluster, "Interface out"=w7193:refnum<class "Interface.lvclass">)  [unwired: 7 in]
                n3267 = call-dynamic "Write Object.vi"("error in (no error)"=w7199, "Object"=w7185, "Interface in"=w7193) -> ("error out"=w7198:errorcluster, "Interface out"=w7192:refnum<class "Interface.lvclass">)  [unwired: 7 in]
                n3268 = call-dynamic "Write Comments.vi"("error in (no error)"=w7198, "Comments"=w7187, "Interface in"=w7192) -> ("error out"=w7179:errorcluster, "Interface out"=w7178:refnum<class "Interface.lvclass">)  [unwired: 7 in]
                n3269 = call-dynamic "Write Observer.vi"("error in (no error)"=w7179, "Observer"=w7184, "Interface in"=w7178) -> ("error out"=w7180:errorcluster, "Interface out"=w7181:refnum<class "Interface.lvclass">)  [unwired: 7 in]
                n3270 = call-dynamic "Write Interface.vi"("error in (no error)"=w7180, "Interface.lvclass"=w7181, "Channel in"=w7195) -> ("error out"=w7173:errorcluster, "Channel out"=w7174:refnum<class "Channel.lvclass">)  [unwired: 7 in]
                n3271 = call-dynamic "Read State Machine.vi"("error in (no error)"=w7173, "Device in"=w7174) -> ("error out"=w7177:errorcluster, "State Machine.lvclass"=w7170:refnum<class "State Machine.lvclass">, "Device out"=w7172:refnum<class "Channel.lvclass">)  [unwired: 7 in]
                n3272 = call "Next State.vi"("error in (no error)"=w7177, "New_State"=12, "State Machine in"=w7170) -> ("error out"=w7176:errorcluster, "State Machine out"=w7169:refnum<class "State Machine.lvclass">)  [unwired: 7 in]
                n3273 = call-dynamic "Write State Machine.vi"("error in (no error)"=w7176, "State Machine.lvclass"=w7169, "Device in"=w7172) -> ("error out"=w7168:errorcluster, "Device out"=w7171:refnum<class "Channel.lvclass">)  [unwired: 7 in]
                n3274 = call-dynamic "Write Channel.vi"("error in (no error)"=w7168, "Channel.lvclass"=w7171, "Acquisition in"=w7190) -> ("error out"=w7188:errorcluster, "Acquisition out"=w7189:refnum<class "Acquisition.lvclass">)  [unwired: 7 in]
                n3275 = call-dynamic "Write AcquisitionC.vi"("error in (no error)"=w7188, "Acquisition.lvclass"=w7189, "S4ACS_GUI in"=w7191) -> ("error out"=w7202:errorcluster, "S4ACS_GUI out"=w7203:refnum<class "S4GUI.lvclass">)  [unwired: 7 in]
              }
              frame #3 {
                # "object"
                # "suffix"
                # "obsType"
                n3276 = call-dynamic "Read AcquisitionD.vi"("error in (no error)"=w7247, "S4ACS_GUI in"=w7248) -> ("error out"=w7240:errorcluster, "Acquisition.lvclass"=w7239:refnum<class "Acquisition.lvclass">, "S4ACS_GUI out"=w7234:refnum<class "S4GUI.lvclass">)  [unwired: 7 in]
                n3277 = call-dynamic "Read Channel.vi"("error in (no error)"=w7240, "Acquisition in"=w7239) -> ("error out"=w7207:errorcluster, "Channel.lvclass"=w7209:refnum<class "Channel.lvclass">, "Acquisition out"=w7233:refnum<class "Acquisition.lvclass">)  [unwired: 7 in]
                n3278 = local read "Filter4"() -> (w7210:u8)
                n3279 = call-dynamic "Write Filter.vi"("error in (no error)"=w7207, "Filter"=w7210, "Channel in"=w7209) -> ("error out"=w7206:errorcluster, "Channel out"=w7208:refnum<class "Channel.lvclass">)  [unwired: 7 in]
                n3280 = call-dynamic "Read Interface.vi"("error in (no error)"=w7206, "Channel in"=w7208) -> ("error out"=w7225:errorcluster, "Interface.lvclass"=w7226:refnum<class "Interface.lvclass">, "Channel out"=w7238:refnum<class "Channel.lvclass">)  [unwired: 7 in]
                n3281 = call-dynamic "Write Suffix.vi"("error in (no error)"=w7225, "Suffix"=w7244, "Interface in"=w7226) -> ("error out"=w7243:errorcluster, "Interface out"=w7237:refnum<class "Interface.lvclass">)  [unwired: 7 in]
                n3282 = call-dynamic "Write ObsType.vi"("error in (no error)"=w7243, "ObsType"=w7229, "Interface in"=w7237) -> ("error out"=w7242:errorcluster, "Interface out"=w7236:refnum<class "Interface.lvclass">)  [unwired: 7 in]
                n3283 = call-dynamic "Write Object.vi"("error in (no error)"=w7242, "Object"=w7228, "Interface in"=w7236) -> ("error out"=w7241:errorcluster, "Interface out"=w7235:refnum<class "Interface.lvclass">)  [unwired: 7 in]
                n3284 = call-dynamic "Write Comments.vi"("error in (no error)"=w7241, "Comments"=w7230, "Interface in"=w7235) -> ("error out"=w7224:errorcluster, "Interface out"=w7223:refnum<class "Interface.lvclass">)  [unwired: 7 in]
                n3285 = call-dynamic "Write Observer.vi"("error in (no error)"=w7224, "Observer"=w7227, "Interface in"=w7223) -> ("error out"=w7219:errorcluster, "Interface out"=w7218:refnum<class "Interface.lvclass">)  [unwired: 7 in]
                n3286 = call-dynamic "Write Interface.vi"("error in (no error)"=w7219, "Interface.lvclass"=w7218, "Channel in"=w7238) -> ("error out"=w7214:errorcluster, "Channel out"=w7217:refnum<class "Channel.lvclass">)  [unwired: 7 in]
                n3287 = call-dynamic "Read State Machine.vi"("error in (no error)"=w7214, "Device in"=w7217) -> ("error out"=w7222:errorcluster, "State Machine.lvclass"=w7212:refnum<class "State Machine.lvclass">, "Device out"=w7216:refnum<class "Channel.lvclass">)  [unwired: 7 in]
                n3288 = call "Next State.vi"("error in (no error)"=w7222, "New_State"=12, "State Machine in"=w7212) -> ("error out"=w7221:errorcluster, "State Machine out"=w7211:refnum<class "State Machine.lvclass">)  [unwired: 7 in]
                n3289 = call-dynamic "Write State Machine.vi"("error in (no error)"=w7221, "State Machine.lvclass"=w7211, "Device in"=w7216) -> ("error out"=w7213:errorcluster, "Device out"=w7215:refnum<class "Channel.lvclass">)  [unwired: 7 in]
                n3290 = call-dynamic "Write Channel.vi"("error in (no error)"=w7213, "Channel.lvclass"=w7215, "Acquisition in"=w7233) -> ("error out"=w7231:errorcluster, "Acquisition out"=w7232:refnum<class "Acquisition.lvclass">)  [unwired: 7 in]
                n3291 = call-dynamic "Write AcquisitionD.vi"("error in (no error)"=w7231, "Acquisition.lvclass"=w7232, "S4ACS_GUI in"=w7234) -> ("error out"=w7245:errorcluster, "S4ACS_GUI out"=w7246:refnum<class "S4GUI.lvclass">)  [unwired: 7 in]
              }
            }
          }
          frame Enabled {
          }
        }
      }
      event "object suffix", "dflat suffix", "sflat suffix", "dark suffix", "zero suffix", "focus suffix": Value Change {
        w7251 = T33 0 items=["both", "start of string", "end of string"] ("location (both)")
        # "Remove todos <\\n> e <space> do sufixo:"
        n3292 = event-data() -> ("NewVal"=w7265:string)  [unwired: 1 in, 5 out]
        n3293 = To Lower Case(string=w7265) -> (all lower case string=w7264:string)
        n3294 = call <vilib>:"Trim Whitespace.vi"("string"=w7264, "location (both)"=w7251) -> ("trimmed string"=w7263:string)
        n3295 = Search and Replace String(replace all?=TRUE ("replace all? (F)"), input string=w7263, search string="\n") -> (result string=w7262:string)  [unwired: 5 in, 3 out]
        n3296 = call <vilib>:"Space Constant.vi"() -> ("String"=w7260:string)
        n3297 = Search and Replace String(replace all?=TRUE ("replace all? (F)"), input string=w7262, search string=w7260) -> (result string=w7256:string)  [unwired: 5 in, 3 out]
        n3298 = case shown="\"DARK\"" w7257 {
          tunnel: w7256 -> [w7479 w7486 w7491 w7496 w7501 w7506]
          tunnel: w7255 -> [w7483 w7488 w7493 w7498 w7503 w7508]
          tunnel: w7254 -> [w7481 w7487 w7492 w7497 w7502 w7507]
          tunnel: [w7482 w7485 w7490 w7494 w7499 w7504] -> w7253
          tunnel: [w7480 w7484 w7489 w7495 w7500 w7505] -> w7252
          frame "OBJECT", Default {
            n3299 = local write "object suffix"(w7479) -> ()
            n3300 = call-dynamic "Write object_suffix.vi"("error in (no error)"=w7481, "object"=w7479, "S4GUI in"=w7483) -> ("error out"=w7480:errorcluster, "S4GUI out"=w7482:refnum<class "S4GUI.lvclass">)  [unwired: 7 in]
          }
          frame "DFLAT" {
            n3301 = local write "dflat suffix"(w7486) -> ()
            n3302 = call-dynamic "Write dflat_suffix.vi"("error in (no error)"=w7487, "dflat"=w7486, "S4GUI in"=w7488) -> ("error out"=w7484:errorcluster, "S4GUI out"=w7485:refnum<class "S4GUI.lvclass">)  [unwired: 7 in]
          }
          frame "SFLAT" {
            n3303 = local write "sflat suffix"(w7491) -> ()
            n3304 = call-dynamic "Write sflat_suffix.vi"("error in (no error)"=w7492, "sflat"=w7491, "S4GUI in"=w7493) -> ("error out"=w7489:errorcluster, "S4GUI out"=w7490:refnum<class "S4GUI.lvclass">)  [unwired: 7 in]
          }
          frame "DARK" {
            n3305 = local write "dark suffix"(w7496) -> ()
            n3306 = call-dynamic "Write dark_suffix.vi"("error in (no error)"=w7497, "dark"=w7496, "S4GUI in"=w7498) -> ("error out"=w7495:errorcluster, "S4GUI out"=w7494:refnum<class "S4GUI.lvclass">)  [unwired: 7 in]
          }
          frame "ZERO" {
            n3307 = local write "zero suffix"(w7501) -> ()
            n3308 = call-dynamic "Write zero_suffix.vi"("error in (no error)"=w7502, "zero"=w7501, "S4GUI in"=w7503) -> ("error out"=w7500:errorcluster, "S4GUI out"=w7499:refnum<class "S4GUI.lvclass">)  [unwired: 7 in]
          }
          frame "FOCUS" {
            n3309 = local write "focus suffix"(w7506) -> ()
            n3310 = call-dynamic "Write focus_suffix.vi"("error in (no error)"=w7507, "focus"=w7506, "S4GUI in"=w7508) -> ("error out"=w7505:errorcluster, "S4GUI out"=w7504:refnum<class "S4GUI.lvclass">)  [unwired: 7 in]
          }
        }
        n3311 = disable-structure shown="Enabled" {
          disable-tunnel: w7271 -> [w7280 _]
          disable-tunnel: w7270 -> [w7279 _]
          disable-tunnel: w7269 -> [w7278 _]
          disable-tunnel: w7268 -> [w7277 _]
          disable-tunnel: [w7276 w7478] -> w7267
          disable-tunnel: [w7275 w7477] -> w7266
          disable-tunnel: w7256 -> [w7274 _]
          disable-tunnel: w7253 -> [w7273 w7478]
          disable-tunnel: w7252 -> [w7272 w7477]
          frame Disabled {
            n3312 = stacked-sequence {
              seq-local: [w7302 _ _ _] -> [_ w7366 _ _]
              seq-local: [w7301 _ _ _] -> [_ w7365 _ _]
              seq-local: [_ w7364 _ _] -> [_ _ w7415 _]
              seq-local: [_ w7363 _ _] -> [_ _ w7414 _]
              seq-local: [_ _ w7413 _] -> [_ _ _ w7464]
              seq-local: [_ _ w7412 _] -> [_ _ _ w7463]
              tunnel: w7272 -> [w7314 _ _ _]
              tunnel: w7273 -> [w7313 _ _ _]
              tunnel: [_ _ _ w7462] -> w7276
              tunnel: [_ _ _ w7461] -> w7275
              tunnel: w7274 -> [w7300 w7362 w7411 w7460]
              tunnel: w7279 -> [w7299 w7361 w7397 w7446]
              tunnel: w7277 -> [w7298 w7347 w7396 w7445]
              tunnel: w7280 -> [w7297 w7346 w7395 w7444]
              tunnel: w7278 -> [w7296 w7345 w7394 w7443]
              frame #0 {
                # "observer"
                # "comment"
                # "object"
                # "suffix"
                # "obsType"
                n3313 = call-dynamic "Read AcquisitionA.vi"("error in (no error)"=w7314, "S4ACS_GUI in"=w7313) -> ("error out"=w7312:errorcluster, "Acquisition.lvclass"=w7311:refnum<class "Acquisition.lvclass">, "S4ACS_GUI out"=w7306:refnum<class "S4GUI.lvclass">)  [unwired: 7 in]
                n3314 = call-dynamic "Read Channel.vi"("error in (no error)"=w7312, "Acquisition in"=w7311) -> ("error out"=w7282:errorcluster, "Channel.lvclass"=w7285:refnum<class "Channel.lvclass">, "Acquisition out"=w7305:refnum<class "Acquisition.lvclass">)  [unwired: 7 in]
                n3315 = local read "Filter1"() -> (w7283:u8)
                n3316 = call-dynamic "Write Filter.vi"("error in (no error)"=w7282, "Filter"=w7283, "Channel in"=w7285) -> ("error out"=w7281:errorcluster, "Channel out"=w7284:refnum<class "Channel.lvclass">)  [unwired: 7 in]
